vi "HEAD.vi"(6 "timeout (10000)":i32=10000, 8 "error in (no error)":errorcluster, 10 "url":string, 11 "HTTP Client Advanced in":refnum<class "HTTP Client Advanced.lvclass">) -> (0 "error out":errorcluster, 2 "headers":string, 3 "HTTP Client Advanced out":refnum<class "HTTP Client Advanced.lvclass">)   [LabVIEW 2021, in "HTTP Client Advanced.lvclass"]
uses:
  HTTP Client Advanced.lvclass
  HTTP Client Advanced.lvclass/HTTP Client Advanced.ctl
  <vilib>/NI/Advanced HTTP Client/Session.lvclass
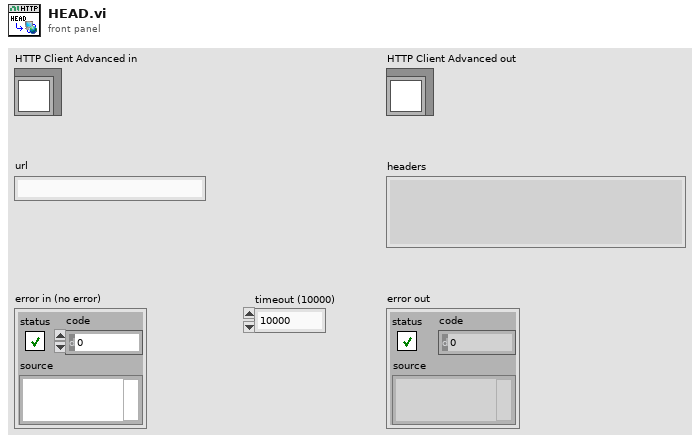
[diagram p1: front panel]
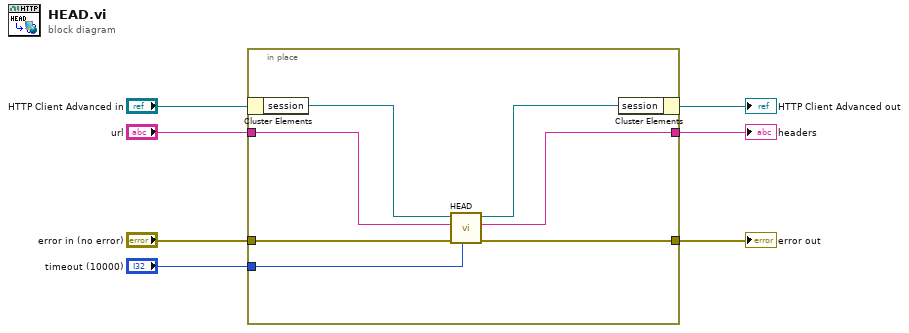
[diagram p0: block diagram]
diagram:
  n1 = in-place {
    in-place-border: "error in (no error)" -> [w14]
    in-place-border: [w13] -> w5
    in-place-border: "url" -> [w10]
    in-place-border: "timeout (10000)" -> [w9]
    in-place-border: [w8] -> w2
    n2 = in-place-cluster #1("HTTP Client Advanced in") -> ("session"=w12:refnum<class "Session.lvclass">)
    n3 = call <vilib>:"HEAD.vi"("timeout"=w9, "error in"=w14, "url"=w10, "session in"=w12) -> ("error out"=w13:errorcluster, "headers"=w8:string, "session out"=w11:refnum<class "Session.lvclass">)  [unwired: 4 in, 1 out]
    n4 = in-place-cluster #1("session"=w11) -> (→"HTTP Client Advanced out":refnum<class "HTTP Client Advanced.lvclass">)
  }
  "error out" <- w5
  "headers" <- w2
